vi "mapped filter.vi"(11 "Path":string) -> (3 "Boolean":bool)   [LabVIEW 2016, in "FPGA RM System Definition API.lvlib"]
uses:
  FPGA-Resource-Manager-APIs/Source/System Definition/FPGA RM System Definition API.lvlib
  Resource Manager/visualizer globals.vi
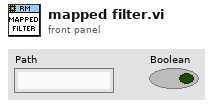
[diagram p1: front panel]
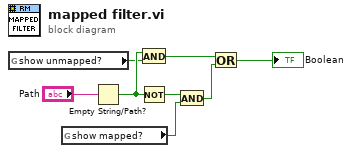
[diagram p0: block diagram]
diagram:
  n1 = global read "visualizer globals.vi" "show unmapped?"() -> (w2:bool)
  n2 = global read "visualizer globals.vi" "show mapped?"() -> (w5:bool)
  n3 = Empty String/Path?(string/path="Path") -> (empty?=w3:bool)
  n4 = And(x=w3, y=w2) -> (x .and. y?=w6:bool)
  n5 = Not(x=w3) -> (.not. x?=w4:bool)
  n6 = And(x=w4, y=w5) -> (x .and. y?=w7:bool)
  n7 = Or(x=w6, y=w7) -> (x .or. y?=→"Boolean":bool)
